vi "NanotecSMCPDDriver.resource data.vi"(0 "VISAresource":refnum<visa-resource-name>, 1 "contollerID":i32=-1, 3 "action":T2(ring), 5 "error in (no error)":errorcluster) -> (14 "VISAresource out":refnum<visa-resource-name>, 15 "contollerID out":i32=-1, 16 "semaphore":T1, 17 "connectionCounter":i32=-1, 19 "error out":errorcluster)   [LabVIEW 2014, in "NanotecSMCPDDriver.lvlib"]
doc: "Functional Global Variable (FGV) storing extended resource proporties. This routine always returns the input value for VISA resource and controllerID. A semaphore reference is provided that is used by the transaction. Please note the following:\n\n- The semaphore is managed by THIS routine.\n- The connection counter is managed by THIS routine\n- Opening and Closing the VISA session must be done somewhere else."
uses:
  NanotecSMCPDDriver.lvlib
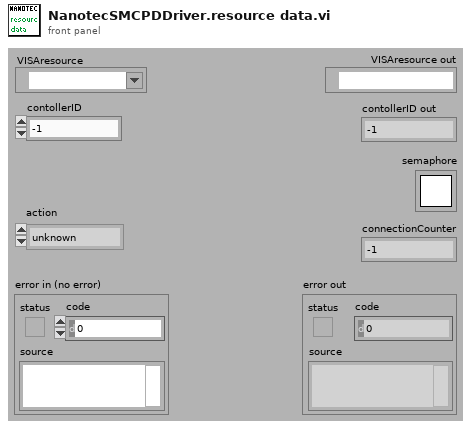
[diagram p1: front panel]
types:
  T1 = typedef "Semaphore RefNum" = refnum<k1>
  T2 = enum16{"unknown", "add", "remove", "get", "cleanup"}
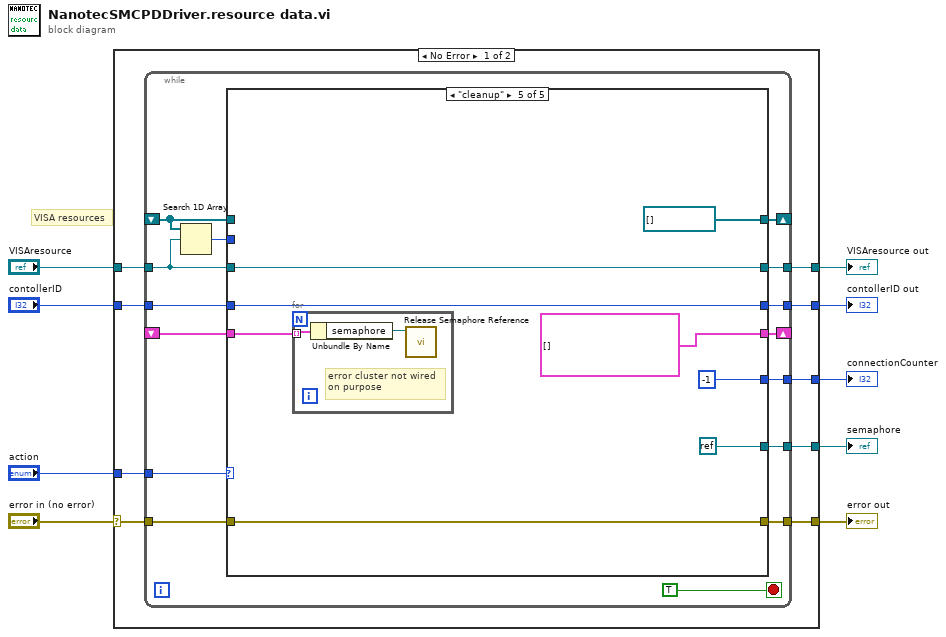
[diagram p0: block diagram]
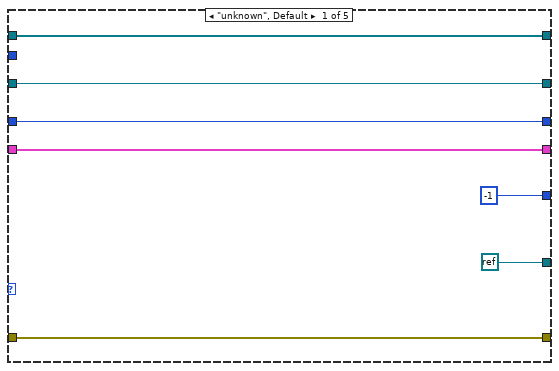
[diagram p2: hidden frame]
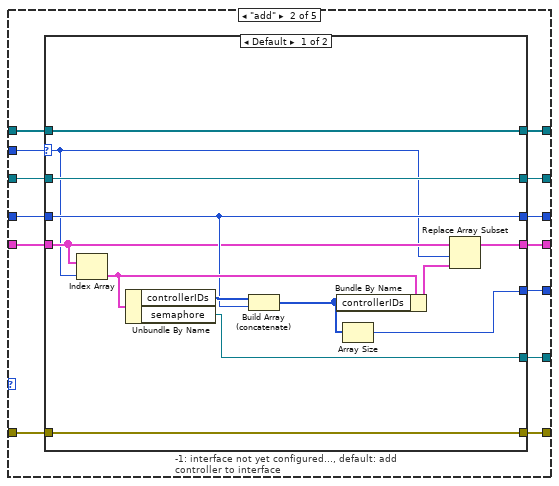
[diagram p3: hidden frame]
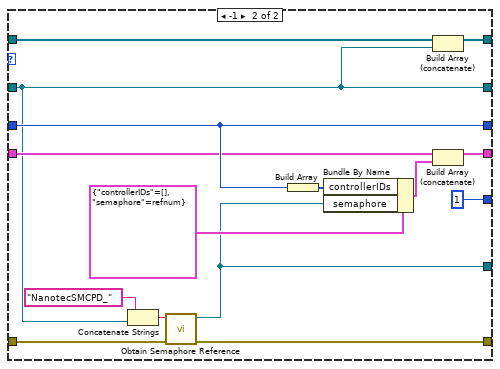
[diagram p4: hidden frame]
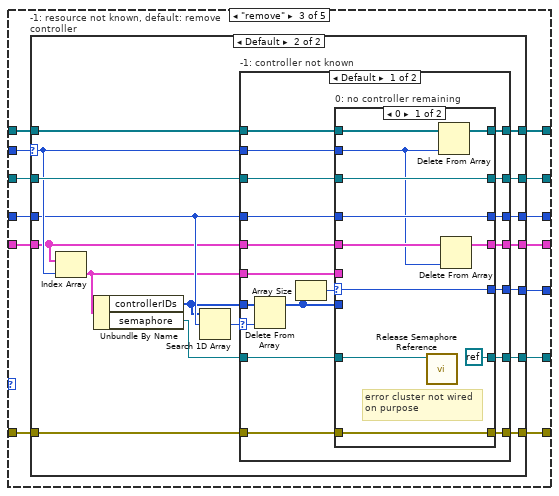
[diagram p5: hidden frame]
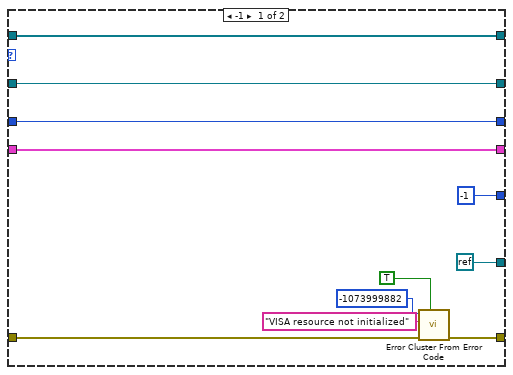
[diagram p6: hidden frame]
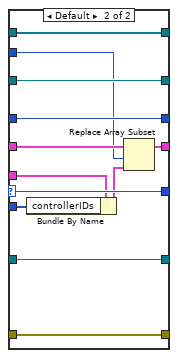
[diagram p7: hidden frame]
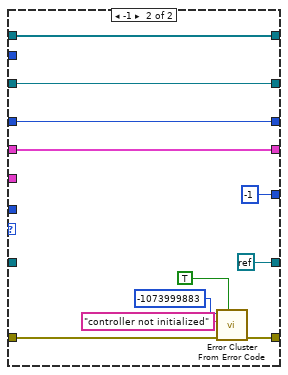
[diagram p8: hidden frame]
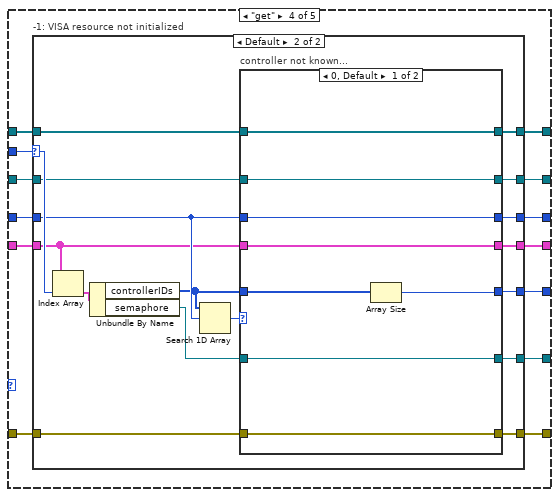
[diagram p9: hidden frame]
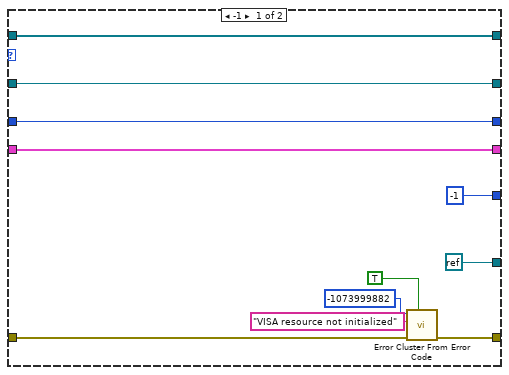
[diagram p10: hidden frame]
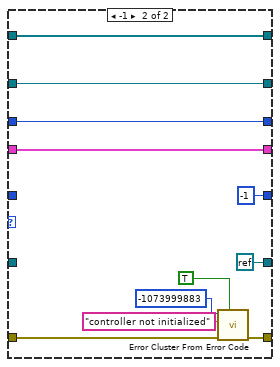
[diagram p11: hidden frame]
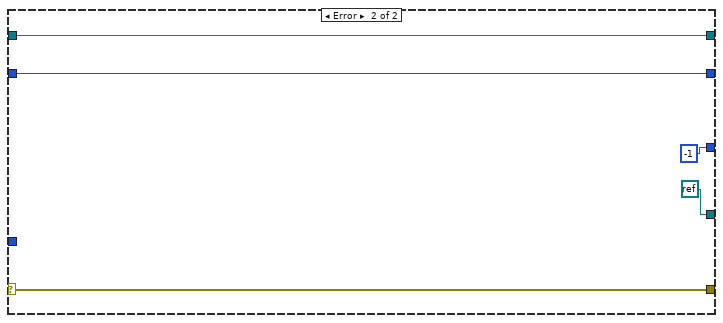
[diagram p12: hidden frame]
diagram:
  # "VISA resources"
  n1 = case shown="No Error" "error in (no error)" {
    selector: "error in (no error)" -> [w18 w246]
    tunnel: [w14 w250] -> w7
    tunnel: "VISAresource" -> [w15 w250]
    tunnel: [w12 w249] -> w5
    tunnel: "contollerID" -> [w13 w249]
    tunnel: [w17 w246] -> w4
    tunnel: "action" -> [w16 _]
    tunnel: [w10 -1] -> w2
    tunnel: [w11 refnum<k0> refnum ("Not a Refnum Constant")] -> w1
    frame No Error {
      n2 = while {
        tunnel: w18 -> [w32]
        tunnel: [w31] -> w17
        tunnel: w16 -> [w30]
        tunnel: w15 -> [w23]
        tunnel: [w22] -> w14
        tunnel: w13 -> [w21]
        tunnel: [w29] -> w12
        shift-right: [w28] -> _
        shift-left: _ -> [w24]
        tunnel: [w27] -> w11
        tunnel: [w26] -> w10
        shift-right: [w19] -> _
        shift-left: _ -> [w20]
        stop <- TRUE stop-if-true
        n3 = Search 1D Array(1D array=w24, element=w23) -> (index of element=w25:i32)  [unwired: 1 in]
        n4 = case shown="\"cleanup\"" w30 {
          tunnel: w32 -> [w39 w53 w91 w181 w238]
          tunnel: [w39 w52 w90 w180 w238] -> w31
          tunnel: w23 -> [w35 w49 w92 w185 w242]
          tunnel: [w35 w43 w86 w184 w242] -> w22
          tunnel: w21 -> [w40 w48 w84 w178 w241]
          tunnel: [w40 w47 w87 w186 w241] -> w29
          tunnel: w24 -> [w38 w50 w94 w183 _]
          tunnel: [w38 w51 w93 w182 refnum<visa-resource-name>[] []] -> w28
          tunnel: [refnum<k0> refnum ("Not a Refnum Constant") w46 w89 w187 refnum<k0> refnum ("Not a Refnum Constant")] -> w27
          tunnel: [-1 w45 w88 w188 -1 ("error code (0)")] -> w26
          tunnel: w25 -> [_ w44 w85 w179 _]
          tunnel: w20 -> [w34 w42 w83 w177 w236]
          tunnel: [w34 w41 w82 w176 cluster{"controllerIDs":i32[], "semaphore":T1}[] []] -> w19
          frame "unknown", Default {
          }
          frame "add" {
            n5 = case "-1: interface not yet configured..., default: add controller to interface" shown="Default" w44 {
              selector: w44 -> [w56 _]
              tunnel: w53 -> [w64 w81]
              tunnel: [w64 w80] -> w52
              tunnel: [w65 w79] -> w51
              tunnel: w50 -> [w65 w78]
              tunnel: w49 -> [w66 w67]
              tunnel: [w66 w67] -> w43
              tunnel: [w60 w72] -> w47
              tunnel: w48 -> [w60 w72]
              tunnel: [w63 w73] -> w46
              tunnel: [w54 1] -> w45
              tunnel: w42 -> [w59 w70]
              tunnel: [w58 w69] -> w41
              frame Default {
                n6 = Index Array(array=w59, index=w56) -> (element=w62:cluster{"controllerIDs":i32[], "semaphore":T1})
                n7 = Unbundle By Name(w62) -> ("controllerIDs"=w61:i32[], "semaphore"=w63:T1)
                n8 = Build Array (concatenate)(w61, w60) -> (w55:i32[])
                n9 = Bundle By Name(cluster=w62, "controllerIDs"=w55) -> (w57:cluster{"controllerIDs":i32[], "semaphore":T1})
                n10 = Array Size(array=w55) -> (size(s)=w54:i32)
                n11 = Replace Array Subset(array=w59, new element=w57, index=w56) -> (w58:cluster{"controllerIDs":i32[], "semaphore":T1}[])
              }
              frame -1 {
                n12 = Concatenate Strings("NanotecSMCPD_", w67) -> (w76:string)
                n13 = call <vilib>:"Obtain Semaphore Reference.vi"("error in (no error)"=w81, "name (unnamed)"=w76) -> ("error out"=w80:errorcluster, "semaphore"=w73:T1)  [unwired: 3 in, 1 out]
                n14 = Build Array(w72) -> (w71:i32[])
                n15 = Bundle By Name(cluster=cluster{"controllerIDs":i32[], "semaphore":T1} {"controllerIDs"=[], "semaphore"=refnum}, "controllerIDs"=w71, "semaphore"=w73) -> (w68:cluster{"controllerIDs":i32[], "semaphore":T1})
                n16 = Build Array (concatenate)(w78, w67) -> (w79:refnum<visa-resource-name>[])
                n17 = Build Array (concatenate)(w70, w68) -> (w69:cluster{"controllerIDs":i32[], "semaphore":T1}[])
              }
            }
          }
          frame "remove" {
            n18 = case "-1: resource not known, default: remove controller" shown="Default" w85 {
              selector: w85 -> [_ w113]
              tunnel: w94 -> [w105 w122]
              tunnel: [w105 w121] -> w93
              tunnel: w92 -> [w104 w117]
              tunnel: [w104 w119] -> w86
              tunnel: w91 -> [w103 w115]
              tunnel: [w102 w114] -> w90
              tunnel: [refnum<k0> refnum ("Not a Refnum Constant") w116] -> w89
              tunnel: [-1 ("error code (0)") w120] -> w88
              tunnel: w84 -> [w96 w112]
              tunnel: [w96 w118] -> w87
              tunnel: w83 -> [w95 w110]
              tunnel: [w95 w109] -> w82
              frame -1 {
                n19 = call <vilib>:"Error Cluster From Error Code.vi"("show call chain? (False)"=TRUE, "error in (no error)"=w103, "error message (\"\")"="VISA resource not initialized" ("error message (\"\")"), "error code (0)"=-1073999882) -> ("error out"=w102:errorcluster)  [unwired: 5 in]
              }
              frame Default {
                n20 = Index Array(array=w110, index=w113) -> (element=w106:cluster{"controllerIDs":i32[], "semaphore":T1})
                n21 = Unbundle By Name(w106) -> ("controllerIDs"=w108:i32[], "semaphore"=w107:T1)
                n22 = Search 1D Array(1D array=w108, element=w112) -> (index of element=w111:i32)  [unwired: 1 in]
                n23 = case "-1: controller not known" shown="Default" w111 {
                  selector: w111 -> [w129 _]
                  tunnel: w122 -> [w141 w165]
                  tunnel: [w140 w165] -> w121
                  tunnel: [w139 -1] -> w120
                  tunnel: [w138 w166] -> w119
                  tunnel: [w137 w167] -> w118
                  tunnel: w117 -> [w136 w166]
                  tunnel: [w135 refnum<k0> refnum ("Not a Refnum Constant")] -> w116
                  tunnel: w115 -> [w134 w173]
                  tunnel: [w133 w172] -> w114
                  tunnel: w113 -> [w132 _]
                  tunnel: w112 -> [w131 w167]
                  tunnel: [w125 w168] -> w109
                  tunnel: w110 -> [w126 w168]
                  tunnel: w108 -> [w130 _]
                  tunnel: w107 -> [w127 _]
                  tunnel: w106 -> [w124 _]
                  frame Default {
                    n24 = Delete From Array(array=w130, index=w129) -> (array with subset deleted=w123:i32[])  [unwired: 1 in, 1 out]
                    n25 = Array Size(array=w123) -> (size(s)=w128:i32)
                    n26 = case "0: no controller remaining" shown="0" w128 {
                      selector: w128 -> [w150 w161]
                      tunnel: w141 -> [w152 w164]
                      tunnel: [w151 w164] -> w140
                      tunnel: w132 -> [w142 w156]
                      tunnel: [w150 w161] -> w139
                      tunnel: [w149 w163] -> w138
                      tunnel: [w148 w159] -> w137
                      tunnel: w136 -> [w149 w163]
                      tunnel: w131 -> [w148 w159]
                      tunnel: [refnum<k0> refnum ("Not a Refnum Constant") w160] -> w135
                      tunnel: w134 -> [w146 w162]
                      tunnel: [w146 w162] -> w133
                      tunnel: w127 -> [w145 w160]
                      tunnel: w126 -> [w144 w158]
                      tunnel: [w143 w157] -> w125
                      tunnel: w124 -> [_ w155]
                      tunnel: w123 -> [_ w154]
                      frame 0 {
                        # "error cluster not wired\non purpose"
                        n27 = call <vilib>:"Release Semaphore Reference.vi"("semaphore"=w145) -> ()  [unwired: 9 in, 2 out]
                        n28 = Delete From Array(array=w152, index=w142) -> (array with subset deleted=w151:refnum<visa-resource-name>[])  [unwired: 1 in, 1 out]
                        n29 = Delete From Array(array=w144, index=w142) -> (array with subset deleted=w143:cluster{"controllerIDs":i32[], "semaphore":T1}[])  [unwired: 1 in, 1 out]
                      }
                      frame Default {
                        n30 = Bundle By Name(cluster=w155, "controllerIDs"=w154) -> (w153:cluster{"controllerIDs":i32[], "semaphore":T1})
                        n31 = Replace Array Subset(array=w158, new element=w153, index=w156) -> (w157:cluster{"controllerIDs":i32[], "semaphore":T1}[])
                      }
                    }
                  }
                  frame -1 {
                    n32 = call <vilib>:"Error Cluster From Error Code.vi"("show call chain? (False)"=TRUE, "error in (no error)"=w173, "error message (\"\")"="controller not initialized" ("error message (\"\")"), "error code (0)"=-1073999883) -> ("error out"=w172:errorcluster)  [unwired: 5 in]
                  }
                }
              }
            }
          }
          frame "get" {
            n33 = case "-1: VISA resource not initialized" shown="Default" w179 {
              selector: w179 -> [_ w216]
              tunnel: [-1 w202] -> w188
              tunnel: [refnum<k0> refnum ("Not a Refnum Constant") w200] -> w187
              tunnel: w178 -> [w192 w211]
              tunnel: [w192 w210] -> w186
              tunnel: w185 -> [w191 w209]
              tunnel: [w191 w208] -> w184
              tunnel: w183 -> [w190 w207]
              tunnel: [w190 w206] -> w182
              tunnel: w181 -> [w196 w213]
              tunnel: [w195 w212] -> w180
              tunnel: [w189 w204] -> w176
              tunnel: w177 -> [w189 w205]
              frame -1 {
                n34 = call <vilib>:"Error Cluster From Error Code.vi"("show call chain? (False)"=TRUE, "error in (no error)"=w196, "error message (\"\")"="VISA resource not initialized" ("error message (\"\")"), "error code (0)"=-1073999882) -> ("error out"=w195:errorcluster)  [unwired: 5 in]
              }
              frame Default {
                n35 = Index Array(array=w205, index=w216) -> (element=w215:cluster{"controllerIDs":i32[], "semaphore":T1})
                n36 = Unbundle By Name(w215) -> ("controllerIDs"=w203:i32[], "semaphore"=w201:T1)
                n37 = Search 1D Array(1D array=w203, element=w211) -> (index of element=w214:i32)  [unwired: 1 in]
                n38 = case "controller not known..." shown="0, Default" w214 {
                  tunnel: w213 -> [w224 w232]
                  tunnel: [w224 w231] -> w212
                  tunnel: w211 -> [w223 w227]
                  tunnel: [w223 w227] -> w210
                  tunnel: w209 -> [w222 w226]
                  tunnel: [w222 w226] -> w208
                  tunnel: w207 -> [w221 w225]
                  tunnel: [w221 w225] -> w206
                  tunnel: w205 -> [w220 w228]
                  tunnel: [w220 w228] -> w204
                  tunnel: w203 -> [w219 _]
                  tunnel: [w218 -1] -> w202
                  tunnel: w201 -> [w217 _]
                  tunnel: [w217 refnum<k0> refnum ("Not a Refnum Constant")] -> w200
                  frame 0, Default {
                    n39 = Array Size(array=w219) -> (size(s)=w218:i32)
                  }
                  frame -1 {
                    n40 = call <vilib>:"Error Cluster From Error Code.vi"("show call chain? (False)"=TRUE, "error in (no error)"=w232, "error message (\"\")"="controller not initialized" ("error message (\"\")"), "error code (0)"=-1073999883) -> ("error out"=w231:errorcluster)  [unwired: 5 in]
                  }
                }
              }
            }
          }
          frame "cleanup" {
            n41 = for {
              tunnel: w236 -> [w245] mode=indexing
              # "error cluster not wired\non purpose"
              n42 = Unbundle By Name(w245) -> ("semaphore"=w244:T1)
              n43 = call <vilib>:"Release Semaphore Reference.vi"("semaphore"=w244) -> ()  [unwired: 9 in, 2 out]
            }
          }
        }
      }
    }
    frame Error {
    }
  }
  "error out" <- w4
  "VISAresource out" <- w7
  "contollerID out" <- w5
  "connectionCounter" <- w2
  "semaphore" <- w1
